vi "Setup CORS.vi"(0 "Web Request in":refnum<class "Web Request.lvclass">) -> (14 "Web Request out":refnum<class "Web Request.lvclass">, 19 "error out":errorcluster)   [LabVIEW 2014]
uses:
  <vilib>/wsapi/Web Request.lvclass
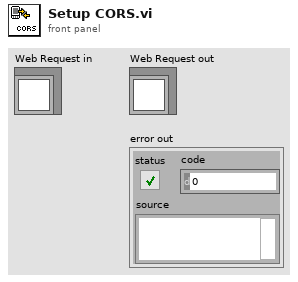
[diagram p1: front panel]
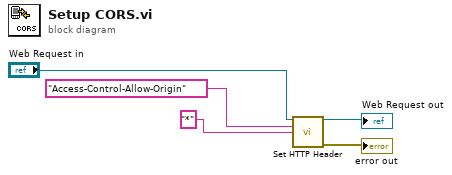
[diagram p0: block diagram]
diagram:
  n1 = call <vilib>:"Set HTTP Header.vi"("LabVIEW Web Service Request"="Web Request in", "header"="Access-Control-Allow-Origin", "header value"="*") -> ("LabVIEW Web Service Request out"=→"Web Request out":refnum<class "Web Request.lvclass">, "error out"=→"error out":errorcluster)  [unwired: 11 in]
